vi "Create Relative Path for Dependency.vi"(0 "old main path":path, 5 "old dependency path":path, 7 "new dir":path, 11 "error in":errorcluster) -> (4 "directory":path, 15 "error out":errorcluster)   [LabVIEW 2021, in "Path Functions.lvlib"]
uses:
  Path Functions.lvlib
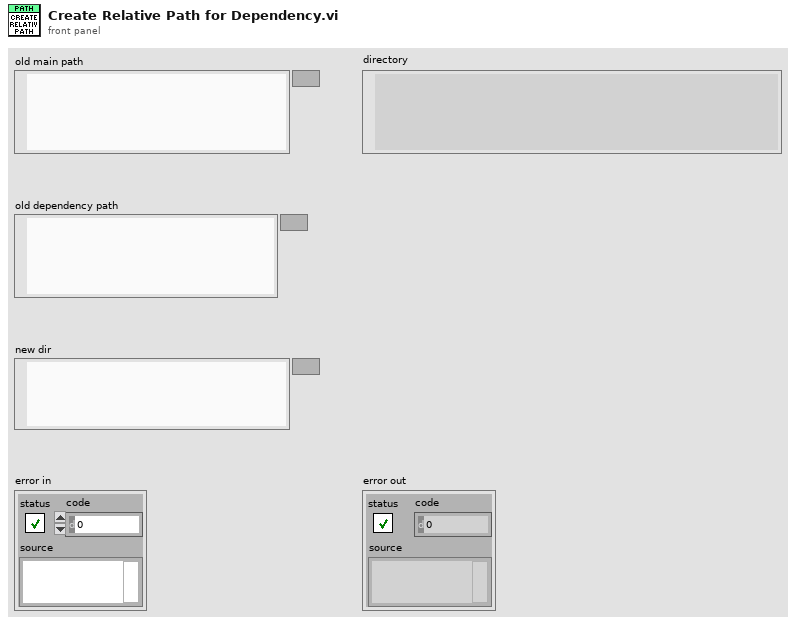
[diagram p1: front panel]
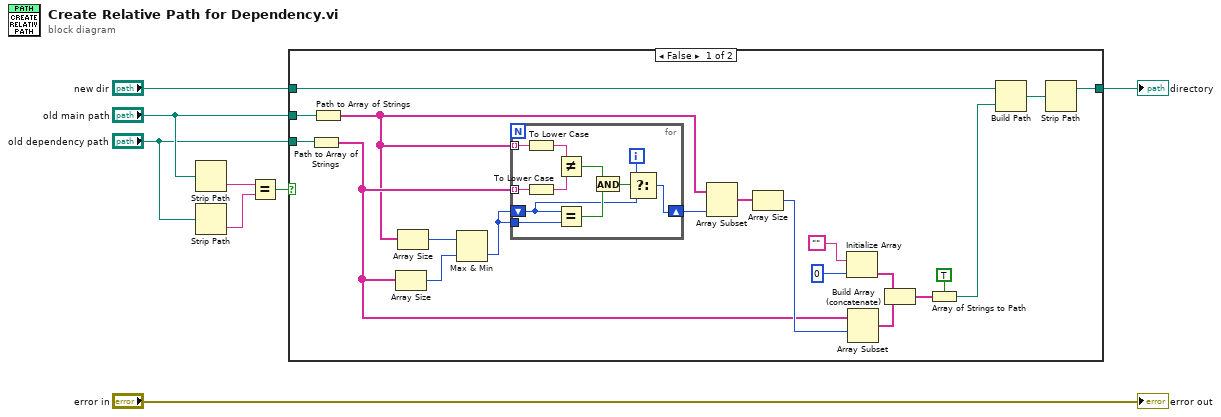
[diagram p0: block diagram]
diagram:
  n1 = Strip Path(path="old main path") -> (name=w6:string)  [unwired: 1 out]
  n2 = Strip Path(path="old dependency path") -> (name=w5:string)  [unwired: 1 out]
  n3 = Equal?(x=w6, y=w5) -> (x = y?=w7:bool)
  n4 = case shown="False" w7 {
    tunnel: "new dir" -> [w11 w40]
    tunnel: [w28 w40] -> w2
    tunnel: "old main path" -> [w27 _]
    tunnel: "old dependency path" -> [w26 _]
    frame False {
      n5 = Path to Array of Strings(0:w26) -> (2:w18:string[])  [unwired: 1 out]
      n6 = Path to Array of Strings(0:w27) -> (2:w9:string[])  [unwired: 1 out]
      n7 = Array Size(array=w18) -> (size(s)=w17:i32)
      n8 = Array Size(array=w9) -> (size(s)=w22:i32)
      n9 = Max & Min(x=w22, y=w17) -> (min(x,y)=w23:i32)  [unwired: 1 out]
      n10 = for {
        tunnel: w9 -> [w39] mode=indexing
        tunnel: w18 -> [w38] mode=indexing
        shift-right: [w31] -> w19
        shift-left: w23 -> [w32]
        tunnel: w23 -> [w37]
        i -> [w33]
        n11 = To Lower Case(string=w39) -> (all lower case string=w30:string)
        n12 = To Lower Case(string=w38) -> (all lower case string=w29:string)
        n13 = Not Equal?(x=w30, y=w29) -> (x != y?=w35:bool)
        n14 = Equal?(x=w32, y=w37) -> (x = y?=w36:bool)
        n15 = And(x=w35, y=w36) -> (x .and. y?=w34:bool)
        n16 = Select(t=w33, s=w34, f=w32) -> (s? t:f=w31:i32)
      }
      n17 = Array Subset(array=w9, length=w19) -> (w13:string[])  [unwired: 1 in]
      n18 = Array Size(array=w13) -> (size(s)=w24:i32)
      n19 = Initialize Array("", 0 ("dimension size")) -> (w20:string[])
      n20 = Array Subset(array=w18, index=w24) -> (w21:string[])  [unwired: 1 in]
      n21 = Build Array (concatenate)(w20, w21) -> (w14:string[])
      n22 = Array of Strings to Path(0:w14, 1:TRUE ("relative")) -> (2:w10:path)
      n23 = Build Path(base path=w11, name or relative path=w10) -> (appended path=w12:path)
      n24 = Strip Path(path=w12) -> (stripped path=w28:path)  [unwired: 1 out]
    }
    frame True {
    }
  }
  "directory" <- w2
  "error out" <- "error in"
